vi "Requests.vi"(8 "error in (no error)":errorcluster, 9 "write enable":bool=TRUE, 11 "TEST in":refnum<class "TEST.lvclass">) -> (0 "error out":errorcluster, 3 "TEST out":refnum<class "TEST.lvclass">)   [LabVIEW 2021, in "TEST.lvclass"]
uses:
  TEST.lvclass
  D:/my_projects/projects/Algorithms/Labview/21/Modbus_v121c/Network Protocol/MB/Modbus Master CR.lvclass
  MB/Modbus Master CR.lvclass/Modbus Master CR.ctl
  Data Model/Device Data Model.lvclass
  MB/Modbus Master CR.lvclass
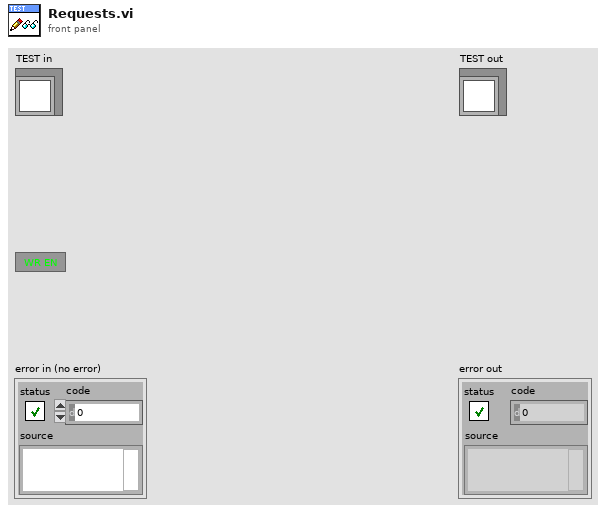
[diagram p1: front panel]
types:
  T1 = typedef "Modbus Master CR.lvclass/N channel.ctl" = cluster{"N DI channel":u16, "N DO channel":u16, "N AI channel":u16, "N AO channel":u16}
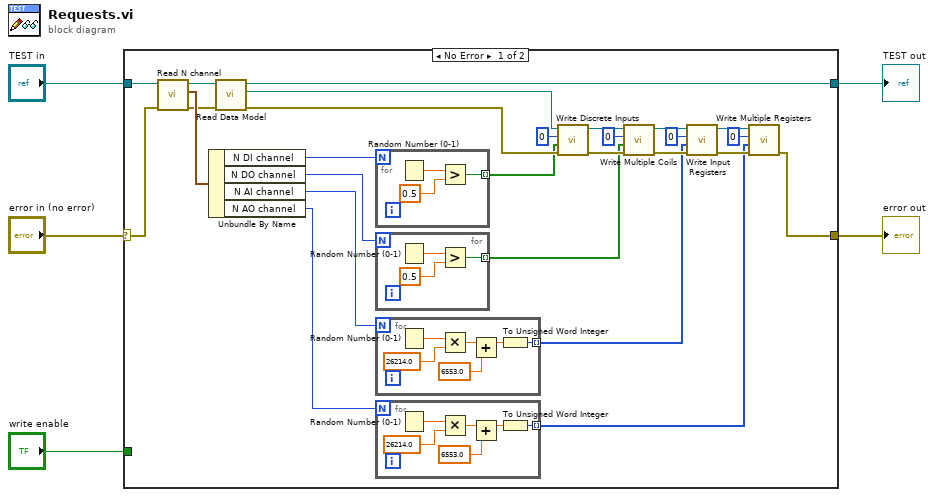
[diagram p0: block diagram]
diagram:
  n1 = case shown="No Error" "error in (no error)" {
    selector: "error in (no error)" -> [w27 w52]
    tunnel: [w7 w52] -> w3
    tunnel: [w25 w51] -> w4
    tunnel: "TEST in" -> [w29 w51]
    tunnel: "write enable" -> [_ _]
    frame No Error {
      n2 = call "Read N channel.vi"("error in (no error)"=w27, "MB_v2 in"=w29) -> ("error out"=w26:errorcluster, "N channel"=w30:T1, "MB_v2 out"=w28:refnum<class "TEST.lvclass">)  [unwired: 7 in]
      n3 = Unbundle By Name(w30) -> ("N DI channel"=w22:u16, "N DO channel"=w21:u16, "N AI channel"=w24:u16, "N AO channel"=w20:u16)
      n4 = call "Read Data Model.vi"("error in (no error)"=w26, "MB_TCP in"=w28) -> ("error out"=w12:errorcluster, "Data Model"=w6:refnum<class "Device Data Model.lvclass">, "MB_TCP out"=w25:refnum<class "TEST.lvclass">)  [unwired: 7 in]
      n5 = for {
        N: w22 -> [_]
        tunnel: [w33] -> w11 mode=indexing
        n6 = Random Number (0-1)() -> (number: 0 to 1=w35:dbl)
        n7 = Greater?(x=w35, y=0.5) -> (0:w33:bool)
      }
      n8 = for {
        N: w21 -> [_]
        tunnel: [w48] -> w10 mode=indexing
        n9 = Random Number (0-1)() -> (number: 0 to 1=w50:dbl)
        n10 = Greater?(x=w50, y=0.5) -> (0:w48:bool)
      }
      n11 = for {
        N: w24 -> [_]
        tunnel: [w44] -> w9 mode=indexing
        n12 = Random Number (0-1)() -> (number: 0 to 1=w47:dbl)
        n13 = Multiply(x=w47, y=26214.0) -> (x*y=w45:dbl)
        n14 = Add(x=w45, y=6553.0) -> (x+y=w43:dbl)
        n15 = To Unsigned Word Integer(number=w43) -> (unsigned 16bit integer=w44:u16)
      }
      n16 = for {
        N: w20 -> [_]
        tunnel: [w38] -> w8 mode=indexing
        n17 = Random Number (0-1)() -> (number: 0 to 1=w41:dbl)
        n18 = Multiply(x=w41, y=26214.0) -> (x*y=w39:dbl)
        n19 = Add(x=w39, y=6553.0) -> (x+y=w37:dbl)
        n20 = To Unsigned Word Integer(number=w37) -> (unsigned 16bit integer=w38:u16)
      }
      n21 = call-dynamic "Write Discrete Inputs.vi"("error in (no error)"=w12, "input values"=w11, "starting address"=u16 0, "Device Data Model in"=w6) -> ("error out"=w14:errorcluster, "Device Data Model out"=w18:refnum<class "Device Data Model.lvclass">)  [unwired: 6 in]
      n22 = call-dynamic "Write Multiple Coils.vi"("error in"=w14, "coils"=w10, "starting address"=u16 0, "device data model in"=w18) -> ("error out"=w13:errorcluster, "device data model out"=w17:refnum<class "Device Data Model.lvclass">)  [unwired: 6 in]
      n23 = call-dynamic "Write Input Registers.vi"("error in (no error)"=w13, "register values"=w9, "starting address"=u16 0, "Device Data Model in"=w17) -> ("error out"=w15:errorcluster, "Device Data Model out"=w16:refnum<class "Device Data Model.lvclass">)  [unwired: 6 in]
      n24 = call-dynamic "Write Multiple Registers.vi"("error in"=w15, "register values"=w8, "starting address"=u16 0, "device data model in"=w16) -> ("error out"=w7:errorcluster)  [unwired: 6 in, 1 out]
    }
    frame Error {
    }
  }
  "error out" <- w3
  "TEST out" <- w4
